vi "Global_CMD_Data Out.vi"() -> ()   [LabVIEW 2020, in "MotionMaster_SubCMD.lvlib"]
uses:
  MotionMaster_SubCMD.lvlib
  Shared Code/TypeDefs/Cluster_MotionMaster Output.ctl
  Shared Code/TypeDefs/Cluster_Pose Positions.ctl
  ENUM_Pose List.ctl
panel:
  out "SubCMD_MotionMaster_Output":T1
  in  "SubCMD_MotionMaster_CycleTime(S)":dbl
  # "The Names of the Data items in the Global Variable MUST describe who the Single Writer is\nFor CMD Globals the the naming convention is\n   \nCMD_Lib Name_Data Name\n\nExamples:\nCMD_RobotArm_Mode\nCMD_AutoTrack_Mode"
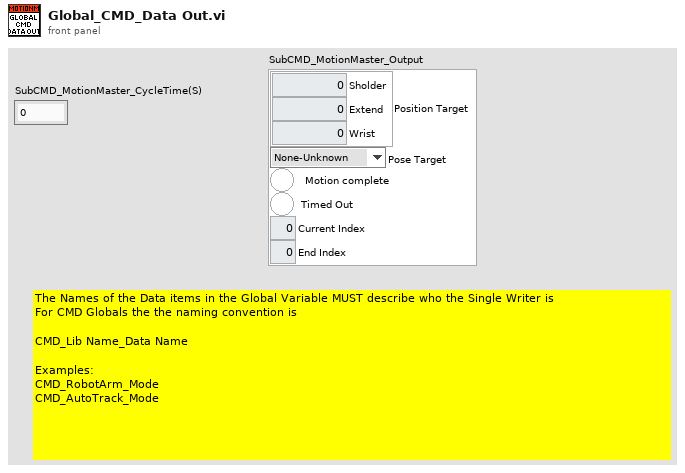
[diagram p1: front panel]
types:
  T1 = typedef "Cluster_MotionMaster Output.ctl" = cluster{"Position Target":T2, "Pose Target":T3, "Motion complete":bool, "Timed Out":bool, "Current Index":i32, "End Index":i32}
  T2 = typedef "Cluster_Pose Positions.ctl" = cluster{"Sholder":i32, "Extend":i32, "Wrist":i32}
  T3 = typedef "MotionMaster_SubCMD.lvlib/ENUM_Pose List.ctl" = enum16{"None-Unknown", "Intake", "Score High", "Score Mid", "Safe Position", "Home Pos"}
diagram:
